vi "Get Session.vi"(8 "error in (no error)":errorcluster, 11 "FTP in":refnum<class "FTP.lvclass">) -> (0 "error out":errorcluster, 2 "ftp session":T1, 3 "FTP out":refnum<class "FTP.lvclass">)   [LabVIEW 2015, in "RT Management.lvlib" / "FTP.lvclass"]
uses:
  FTP.lvclass
  <vilib>/FTP/ftp0.llb/FTP Session.ctl
  FTP.lvclass/FTP.ctl
  <vilib>/FTP/NI_FTP.lvlib
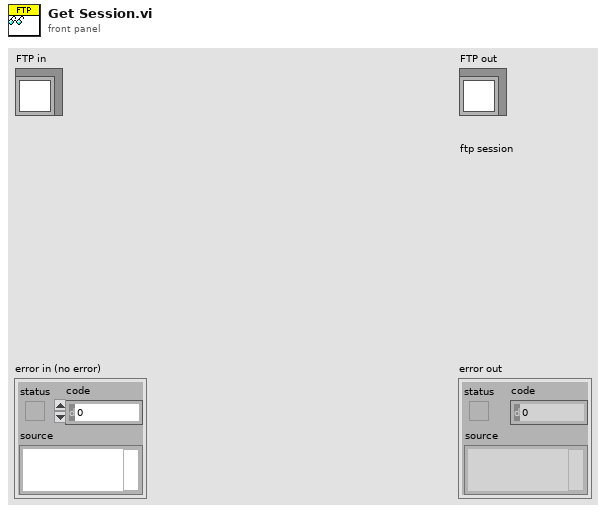
[diagram p1: front panel]
types:
  T1 = typedef "NI_FTP.lvlib/FTP Session.ctl" = refnum<k5>
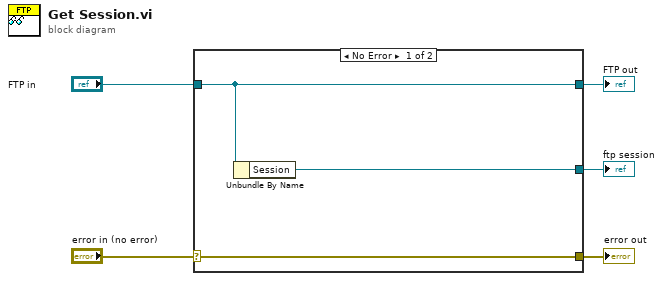
[diagram p0: block diagram]
diagram:
  n1 = case shown="No Error" "error in (no error)" {
    selector: "error in (no error)" -> [w8 w9]
    tunnel: [w8 w9] -> w4
    tunnel: [w7 w10] -> w2
    tunnel: "FTP in" -> [w7 w10]
    tunnel: [w6 _] -> w1
    frame No Error {
      n2 = Unbundle By Name(w7) -> ("Session"=w6:T1)
    }
    frame Error {
    }
  }
  "error out" <- w4
  "FTP out" <- w2
  "ftp session" <- w1
